vi "BUFMGR_Create_Buffer.vi"(0 "Buffer Name":string, 5 "Size in Bytes":u64, 11 "error in (no error)":errorcluster) -> (4 "pointer to buff":u64 format="%.0x", 6 "Size in Bytes out":u64, 15 "error out":errorcluster)   [LabVIEW 2016]
uses:
  c/lib/libbuf.so
panel:
  out "err":i32
  in  "err in":i32
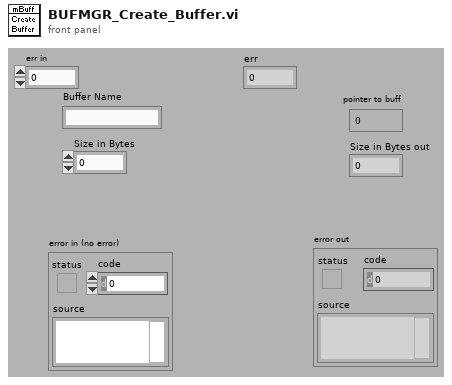
[diagram p1: front panel]
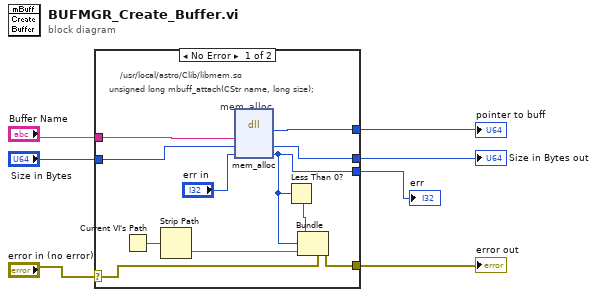
[diagram p0: block diagram]
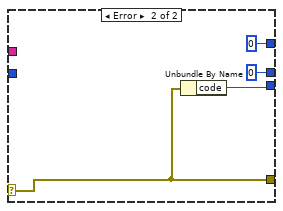
[diagram p2: hidden frame]
diagram:
  n1 = case shown="No Error" "error in (no error)" {
    selector: "error in (no error)" -> [w11 w20]
    tunnel: "Buffer Name" -> [w18 _]
    tunnel: [w13 u32 0] -> w6
    tunnel: "Size in Bytes" -> [w17 _]
    tunnel: [w16 0 ("size")] -> w4
    tunnel: [w15 w20] -> w3
    tunnel: [w9 w19] -> w1
    frame No Error {
      # "/usr/local/astro/Clib/libmem.so"
      # "unsigned long mbuff_attach(CStr name, long size);"
      # "mem_alloc"
      n2 = Current VI's Path() -> (path=w12:path)
      n3 = Strip Path(path=w12) -> (name=w8:string)  [unwired: 1 out]
      n4 = dll-call lib="home/simager/panview/PAN/Modules/buffermgr/private/c/lib/libbuf.so" fn="mem_alloc"("name"=w18, "size"=w17, "err"="err in") -> ("return type"=w13:u64, "size"=w16:u64, "err"=w9:i32)  [unwired: 4 in, 2 out]
      n5 = Less Than 0?(x=w9) -> (x < 0?=w14:bool)
      n6 = Bundle(cluster=w11, "status"=w14, "code"=w9, "source"=w8) -> (w15:errorcluster)
    }
    frame Error {
      n7 = Unbundle By Name(w20) -> ("code"=w19:i32)
    }
  }
  "error out" <- w3
  "pointer to buff" <- w6
  "Size in Bytes out" <- w4
  "err" <- w1
